vi "Tool LEIN m SIC Controller STAT 2 reply.vi"(11 "error in (no error)":errorcluster) -> (4 "notifier out":refnum<notifier>, 15 "error out":errorcluster)   [LabVIEW 2011]
uses:
  LEINmaster/Nodes/STAT2 data carrier type aware.ctl
  List of tools.ctl
  Stroker/Stat def/Stroker system stat2.ctl
  LEINmaster/Nodes/Controller local stat2.ctl
  LEINmaster/Nodes/pressure stat2.ctl
  LEINmaster/Nodes/solonoid stat2.ctl
  LEINmaster/Nodes/PSU stat2.ctl
  LEINmaster/Nodes/tensionsub stat2.ctl
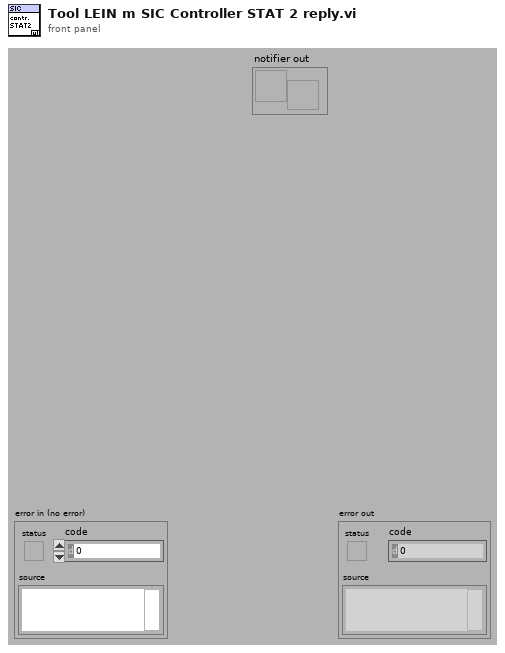
[diagram p1: front panel]
types:
  T1 = typedef "STAT2 data carrier type aware.ctl" = cluster{"Tool":T2, "Data":variant}
  T2 = typedef "List of tools.ctl" = enum16{"Stroker", "Driller", "Tractor"}
  T3 = typedef "Stroker system stat2.ctl" = cluster{"Controller local":T4, "pressure 1":T5, "pressure 2":T5, "solonoid":T6, "PSU":T7, "Tension Sub 1":T8, "Tension Sub 2":T8}
  T4 = typedef "Controller local stat2.ctl" = cluster{"sys register":u16, "temperature":u16, "Input voltage":u16, "Input Current":u16, "Accelerometer ch0":u16, "Accelerometer ch1":u16, "Accelerometer ch2":u16, "Relay status":u8, "GPIO values":u8, "Sensor 1":i32, "Sensor 2":i32, "NA":u8, "High G monitoring":u8}
  T5 = typedef "pressure stat2.ctl" = cluster{"sys register":u16, "temperature":u16, "Pressure":u16, "osctun":u8}
  T6 = typedef "solonoid stat2.ctl" = cluster{"sys register":u16, "temperature":u16, "Position":i16, "monitor state":u8, "valve status":u8}
  T7 = typedef "PSU stat2.ctl" = cluster{"sys register":u16, "temperature":u16, "HV Voltage in":u16, "Main Voltage out":u16, "Main Current out":u16}
  T8 = typedef "tensionsub stat2.ctl" = cluster{"sys register":u16, "temperature":u16, "Tension":i16, "osctun":u8}
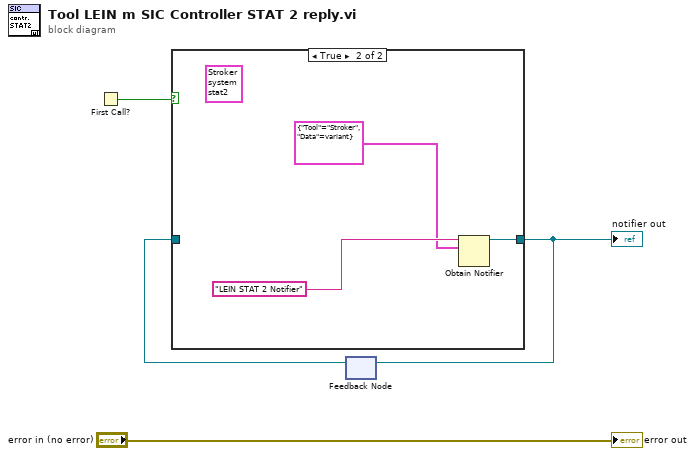
[diagram p0: block diagram]
diagram:
  n1 = First Call?() -> (First Call?: T/F=w3:bool)
  n2 = feedback #1() -> (w1:refnum<notifier>)  [unwired: 1 in]
  n3 = case shown="True" w3 {
    tunnel: [w5 w7] -> w2
    tunnel: w1 -> [w5 _]
    frame False {
    }
    frame True {
      (unwired) T3 {"Controller local"={"sys register"=0, "temperature"=0, "Input voltage"=0, "Input Current"=0, "Accelerometer ch0"=0, "Accelerometer ch1"=0, "Accelerometer ch2"=0, "Relay status"=0, "GPIO values"=0, "Sensor 1"=0, "Sensor 2"=0, "NA"=0, "High G monitoring"=0}, "pressure 1"={"sys register"=0, "temperature"=0, "Pressure"=0, "osctun"=0}, "pressure 2"={"sys register"=0, "temperature"=0, "Pressure"=0, "osctun"=0}, "solonoid"={"sys register"=0, "temperature"=0, "Position"=0, "monitor state"=0, "valve status"=0}, "PSU"={"sys register"=0, "temperature"=0, "HV Voltage in"=0, "Main Voltage out"=0, "Main Current out"=0}, "Tension Sub 1"={"sys register"=0, "temperature"=0, "Tension"=0, "osctun"=0}, "Tension Sub 2"={"sys register"=0, "temperature"=0, "Tension"=0, "osctun"=0}} ("system stat2")
      n4 = Obtain Notifier(name (unnamed)="LEIN STAT 2 Notifier", notification data type=T1 {"Tool"=enum."Stroker", "Data"=variant}) -> (notifier out=w7:refnum<notifier>)  [unwired: 2 in, 2 out]
    }
  }
  "notifier out" <- w2
  n5 = feedback-in #1(w2) -> ()
  "error out" <- "error in (no error)"
